vi "Check New QControl Information.vi"(8 "error in (no error)":errorcluster, 11 "QControl Creation in":refnum<class "QControl Creation.lvclass">) -> (0 "error out":errorcluster, 3 "QControl Creation (dup)":refnum<class "QControl Creation.lvclass">)   [LabVIEW 2015, in "QControl Creation.lvclass"]
doc: "<b> </b> <b> </b>\n©2016 Q Software Innovations, LLC (QSI)\nwritten by Quentin Alldredge\nproduced in LabVIEW 2015\n\nsupport@qsoftwareinnovations.com\nwww.qsoftwareinnovations.com\n\nAll rights reserved.\n\nRedistribution and use in source and binary forms, with or without modification, are permitted provided that the following conditions are met:\n\n * Redistributions of source code must retain the above copyright notice, this list of conditions and the following disclaimer.\n * Redistributions in binary form must reproduce the above copyright notice, this list of conditions and the following disclaimer in the documentation and/or other materials provided with the distribution.\n * Neither the name of Q Software Innovations, LLC. nor the names of its contributors may be used to endorse or promote products derived from this software without specific prior written permission.\n\nTHIS SOFTWARE IS PROVIDED BY THE COPYRIGHT HOLDERS AND CONTRIBUTORS \"AS IS\" AND ANY EXPRESS OR IMPLIED WARRANTIES, INCLUDING, BUT NOT LIMITED TO, THE IMPLIED WARRANTIES OF MERCHANTABILITY AND FITNESS FOR A PARTICULAR PURPOSE ARE DISCLAIMED. IN NO EVENT SHALL THE COPYRIGHT OWNER OR CONTRIBUTORS BE LIABLE FOR ANY DIRECT, INDIRECT, INCIDENTAL, SPECIAL, EXEMPLARY, OR CONSEQUENTIAL DAMAGES (INCLUDING, BUT NOT LIMITED TO, PROCUREMENT OF SUBSTITUTE GOODS OR SERVICES; LOSS OF USE, DATA, OR PROFITS; OR BUSINESS INTERRUPTION) HOWEVER CAUSED AND ON ANY THEORY OF LIABILITY, WHETHER IN CONTRACT, STRICT LIABILITY, OR TORT (INCLUDING NEGLIGENCE OR OTHERWISE) ARISING IN ANY WAY OUT OF THE USE OF THIS SOFTWARE, EVEN IF ADVISED OF THE POSSIBILITY OF SUCH DAMAGE."
uses:
  QControl Creation.lvclass
  QControl Creation.lvclass/QControl Creation.ctl
  New QControl Info/New QControl Info.lvclass
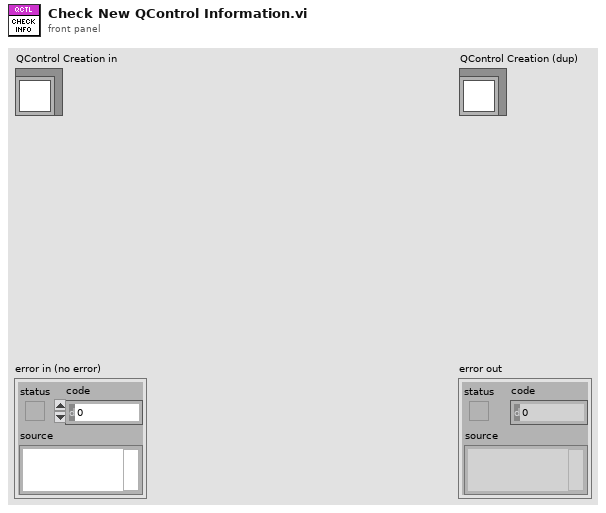
[diagram p1: front panel]
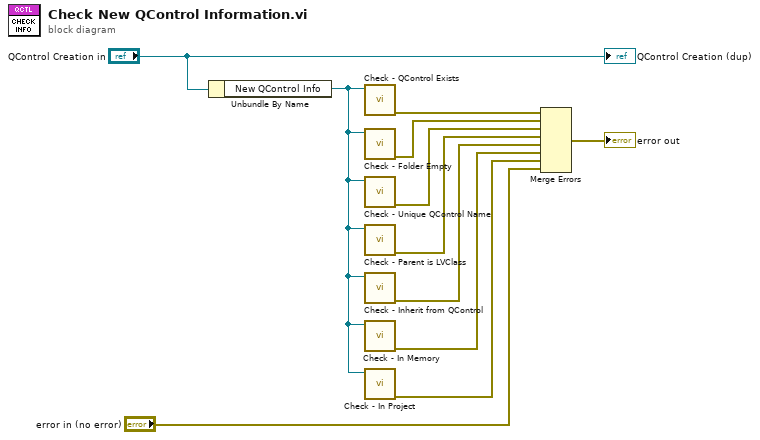
[diagram p0: block diagram]
diagram:
  n1 = Unbundle By Name("QControl Creation in") -> ("New QControl Info"=w1:refnum<data-value>)
  n2 = call "Check - QControl Exists.vi"("New QControl Info"=w1) -> ("error out"=w7:errorcluster)  [unwired: 10 in]
  n3 = call "Check - Folder Empty.vi"("New QControl Info"=w1) -> ("error out"=w8:errorcluster)  [unwired: 10 in]
  n4 = call "Check - Unique QControl Name.vi"("New QControl Info"=w1) -> ("error out"=w5:errorcluster)  [unwired: 10 in]
  n5 = call "Check - Parent is LVClass.vi"("New QControl Info"=w1) -> ("error out"=w4:errorcluster)  [unwired: 10 in]
  n6 = call "Check - Inherit from QControl.vi"("New QControl Info"=w1) -> ("error out"=w10:errorcluster)  [unwired: 10 in]
  n7 = call "Check - In Memory.vi"("New QControl Info"=w1) -> ("error out"=w2:errorcluster)  [unwired: 10 in]
  n8 = call "Check - In Project.vi"("New QControl Info"=w1) -> ("error out"=w3:errorcluster)  [unwired: 10 in]
  n9 = Merge Errors(w7, w8, w5, w4, w10, w2, w3, "error in (no error)") -> (→"error out":errorcluster)
  "QControl Creation (dup)" <- "QControl Creation in"
